vi "ChangeVolume.vi"(8 "error in (no error)":errorcluster, 11 "Menu in":refnum<class "Game.lvclass">) -> (0 "error out":errorcluster, 3 "Menu out":refnum<class "Game.lvclass">)   [LabVIEW 2019, in "RT_Game.lvlib" / "Game.lvclass"]
uses:
  Game.lvclass
  Game.lvclass/Game.ctl
  Engine/ChangeVolumeData.ctl
  Engine/Engine.lvclass
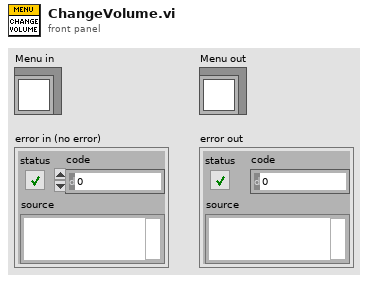
[diagram p1: front panel]
types:
  T1 = cluster{"Controls_1":cluster{"DirectionX":i8, "DirectionY":i8, "Button1":bool, "Button2":bool}, "Controls_2":cluster{"DirectionX":i8, "DirectionY":i8, "Button1":bool, "Button2":bool}, "SystemButton":bool}
  T2 = typedef "RT_Game.lvlib/Engine.lvclass/ChangeVolumeData.ctl" = enum16{"up", "down", "mute"}
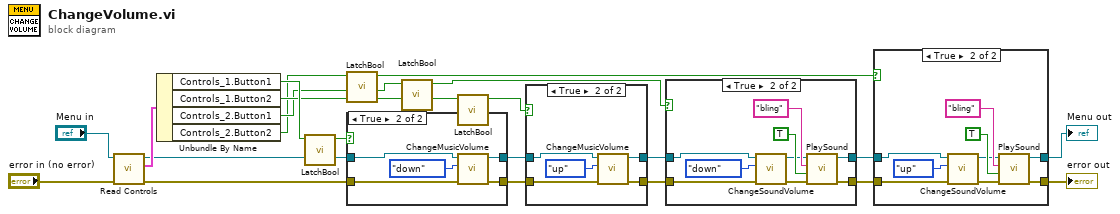
[diagram p0: block diagram]
diagram:
  n1 = call "Read Controls.vi"("error in (no error)"="error in (no error)", "Game in"="Menu in") -> ("error out"=w13:errorcluster, "Controls"=w19:T1, "Game out"=w12:refnum<class "Game.lvclass">)  [unwired: 7 in]
  n2 = Unbundle By Name(w19) -> ("Controls_1.Button1"=w18:bool, "Controls_1.Button2"=w17:bool, "Controls_2.Button1"=w16:bool, "Controls_2.Button2"=w15:bool)
  n3 = call "LatchBool.vi"("Boolean"=w18) -> ("Latched Boolean"=w14:bool)  [unwired: 10 in]
  n4 = call "LatchBool.vi"("Boolean"=w15) -> ("Latched Boolean"=w1:bool)  [unwired: 10 in]
  n5 = case shown="True" w14 {
    tunnel: w13 -> [w22 w28]
    tunnel: w12 -> [w23 w27]
    tunnel: [w22 w24] -> w9
    tunnel: [w23 w25] -> w10
    frame False {
    }
    frame True {
      n6 = call "ChangeMusicVolume.vi"("error in (no error)"=w28, "VolumeData"=ChangeVolumeData."down", "Game in"=w27) -> ("error out"=w24:errorcluster, "Game out"=w25:refnum<class "Game.lvclass">)  [unwired: 7 in]
    }
  }
  n7 = call "LatchBool.vi"("Boolean"=w16) -> ("Latched Boolean"=w2:bool)  [unwired: 10 in]
  n8 = call "LatchBool.vi"("Boolean"=w17) -> ("Latched Boolean"=w11:bool)  [unwired: 10 in]
  n9 = case shown="True" w11 {
    tunnel: w9 -> [w29 w35]
    tunnel: w10 -> [w30 w34]
    tunnel: [w29 w31] -> w7
    tunnel: [w30 w32] -> w8
    frame False {
    }
    frame True {
      n10 = call "ChangeMusicVolume.vi"("error in (no error)"=w35, "VolumeData"=ChangeVolumeData."up", "Game in"=w34) -> ("error out"=w31:errorcluster, "Game out"=w32:refnum<class "Game.lvclass">)  [unwired: 7 in]
    }
  }
  n11 = case shown="True" w2 {
    tunnel: w7 -> [w36 w46]
    tunnel: w8 -> [w37 w40]
    tunnel: [w36 w43] -> w5
    tunnel: [w37 w42] -> w6
    frame False {
    }
    frame True {
      n12 = call "ChangeSoundVolume.vi"("error in (no error)"=w46, "VolumeData"=ChangeVolumeData."down", "Game in"=w40) -> ("error out"=w41:errorcluster, "Game out"=w39:refnum<class "Game.lvclass">)  [unwired: 7 in]
      n13 = call "PlaySound.vi"("error in (no error)"=w41, "Overwrite"=TRUE, "Name"="bling", "Game in"=w39) -> ("error out"=w43:errorcluster, "Game out"=w42:refnum<class "Game.lvclass">)  [unwired: 6 in]
    }
  }
  n14 = case shown="True" w1 {
    tunnel: w5 -> [w47 w57]
    tunnel: w6 -> [w48 w51]
    tunnel: [w47 w54] -> w3
    tunnel: [w48 w53] -> w4
    frame False {
    }
    frame True {
      n15 = call "ChangeSoundVolume.vi"("error in (no error)"=w57, "VolumeData"=ChangeVolumeData."up", "Game in"=w51) -> ("error out"=w52:errorcluster, "Game out"=w50:refnum<class "Game.lvclass">)  [unwired: 7 in]
      n16 = call "PlaySound.vi"("error in (no error)"=w52, "Overwrite"=TRUE, "Name"="bling", "Game in"=w50) -> ("error out"=w54:errorcluster, "Game out"=w53:refnum<class "Game.lvclass">)  [unwired: 6 in]
    }
  }
  "error out" <- w3
  "Menu out" <- w4
